vi "kvCanGetBusStatistics.vi"(0 "Channel Handle (input only)":i32, 5 "error in (no error)":errorcluster) -> (10 "Channel Handle (output only)":i32, 12 "Standard Frame Count":u32, 13 "error out":errorcluster, 14 "Standard Remote Frame Count":u32, 15 "Extended Frame Count":u32, 16 "Extended Remote Frame Count":u32, 17 "Error Frame Count":u32, 18 "Bus Load (%)":dbl min=0.0 max=100.0 step=0.01 format="%.2f", 19 "Overrun Count":u32)   [LabVIEW 2022 SP3]
doc: "The canGetBusStatistics function retrieves the latest bus statistics figures reported by the driver. You request the bus statistics from the driver by calling the canRequestBusStatistics function."
uses:
  canlib32.dll
panel:
  in  "kvCanBusStats (inut only)":T1
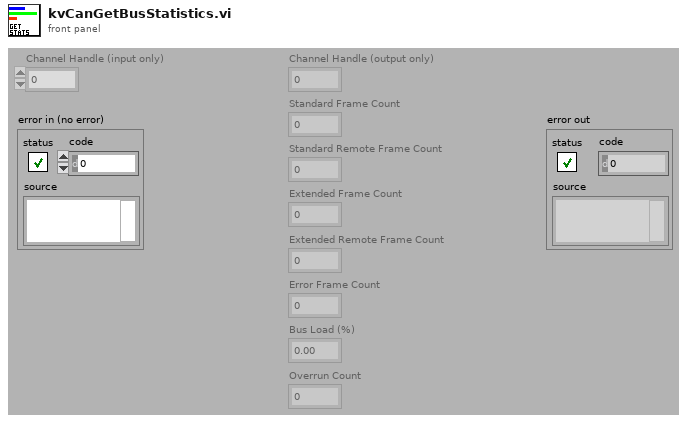
[diagram p1: front panel]
types:
  T1 = cluster{"Standard Frames":i32, "Standard Remote Frames":i32, "Extended Frames":i32, "Extended Remote Frames":i32, "Error Frames":i32, "Bus Load":i32, "Overruns":i32}
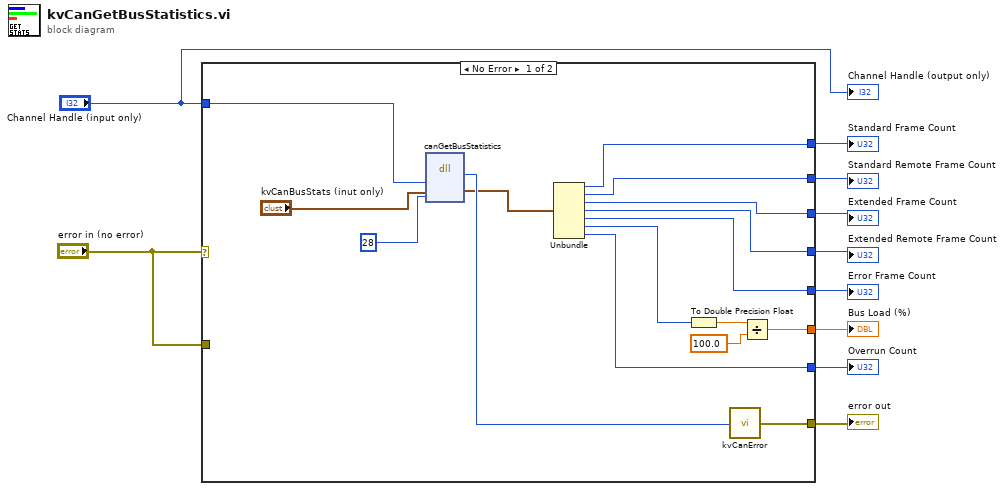
[diagram p0: block diagram]
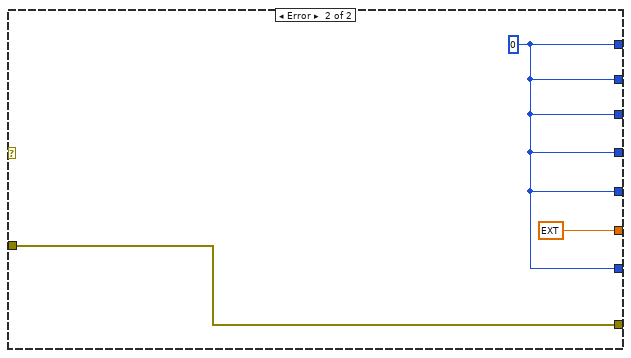
[diagram p2: hidden frame]
diagram:
  n1 = case shown="No Error" "error in (no error)" {
    tunnel: "Channel Handle (input only)" -> [w26 _]
    tunnel: "error in (no error)" -> [_ w29]
    tunnel: [w25 w29] -> w8
    tunnel: [w20 w28] -> w7
    tunnel: [w15 w28] -> w6
    tunnel: [w16 w28] -> w5
    tunnel: [w17 w28] -> w4
    tunnel: [w18 w28] -> w3
    tunnel: [w19 w28] -> w2
    tunnel: [w14 ext 0.0] -> w1
    frame No Error {
      n2 = dll-call lib="canlib32.dll" fn="canGetBusStatistics"("channelHandle"=w26, "kvCanBusStats (inut only)"="kvCanBusStats (inut only)", "bufSize"=28) -> (w24:i32, "kvCanBusStats (inut only)"=w21:T1)  [unwired: 5 in, 2 out]
      n3 = Unbundle(w21) -> ("Standard Frames"=w20:i32, "Standard Remote Frames"=w19:i32, "Extended Frames"=w18:i32, "Extended Remote Frames"=w17:i32, "Error Frames"=w16:i32, "Bus Load"=w13:i32, "Overruns"=w15:i32)
      n4 = To Double Precision Float(number=w13) -> (double precision float=w12:dbl)
      n5 = call "kvCanError.vi"("error code"=w24) -> ("error out"=w25:errorcluster)
      n6 = Divide(x=w12, y=100.0) -> (x/y=w14:dbl)
    }
    frame Error {
      w28 = u32 0
    }
  }
  "error out" <- w8
  "Standard Frame Count" <- w7
  "Standard Remote Frame Count" <- w2
  "Extended Frame Count" <- w3
  "Extended Remote Frame Count" <- w4
  "Error Frame Count" <- w5
  "Bus Load (%)" <- w1
  "Overrun Count" <- w6
  "Channel Handle (output only)" <- "Channel Handle (input only)"
